vi "Global - All RT Loop Stop.vi"() -> ()   [LabVIEW 2013]
panel:
  in  "All RT Loop Stop":bool caption="全部RT循环停止"
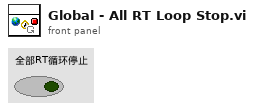
[diagram p1: front panel]
diagram:
